vi "LVITX Format Notes.vi"(1 "Notes":string) -> (0 "String":string)   [LabVIEW 2011]
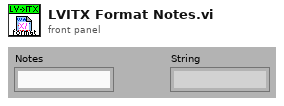
[diagram p1: front panel]
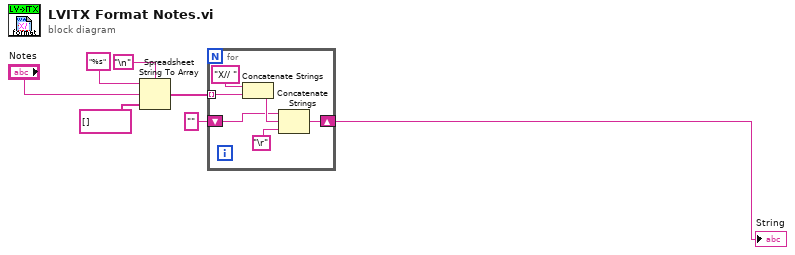
[diagram p0: block diagram]
diagram:
  n1 = Spreadsheet String To Array(delimiter (Tab)="\n", format string="%s", spreadsheet string="Notes", array type (2D Dbl)=string[] [] ("1D Array Names 2")) -> (array=w5:string[])
  n2 = for {
    tunnel: w5 -> [w13] mode=indexing
    shift-right: [w11] -> w6
    shift-left: "" -> [w8]
    n3 = Concatenate Strings("X// " ("string"), w13) -> (w10:string)
    n4 = Concatenate Strings(w8, w10, "\r") -> (w11:string)
  }
  "String" <- w6
